vi "DB - [MasterData].[Material].vi"(0 "connection reference":T5, 1 "DB Connection":T2={"Open"=TRUE, "Close"=TRUE}, 2 "DB - Master Data Material Enum":T4, 3 "Include Inactive":bool=TRUE, 5 "SRTRS.MasterData.SAPMaterial/Material":string="SRTRS.MasterData.SAPMaterial", 7 "[LanguageId]":string, 9 "Update [ShortDescription] to Cluster":bool=TRUE, 11 "error in (no error)":errorcluster, 12 "Clust Refnum":refnum<vi>, 13 "Material File":path=path "c:/temp/Filestream/Test2.jpg", 14 "CmbBox Refnum":refnum<vi>) -> (4 "connection reference":T5, 6 "image data":T1, 8 "ImageFile OK":bool, 10 "Material File":path, 15 "SUMMARY":errorcluster)   [LabVIEW 2013]
uses:
  <vilib>/addons/database/Connection.llb/Conn ObjectReference.ctl
  Controls/DB - Master Data Material Enum.ctl
  Controls/DB - OpenClose.ctl
  <vilib>/picture/picture.llb/imagedata.ctl
  Controls/Global SRTRS.vi
  <vilib>/addons/database/Connection.llb/DB Tools Open Connec (String).vi
  <vilib>/addons/database/Connection.llb/Conn Execute.vi
  <vilib>/addons/database/Recordset.llb/Rec Fetch Recordset Data (R).vi
  <vilib>/addons/database/Recordset.llb/Rec Destroy - Connection.vi
  <vilib>/addons/database/_DB Variant To Data/Database Variant To Data.xnode
  <vilib>/addons/database/NI_Database_API.lvlib
panel:
  in  "SRTRS.MasterData.Material":string="SRTRS.MasterData.Material"
  out "JPG File Error":errorcluster
  out "Property Node Error":errorcluster
  out "Close Error":errorcluster
  out "ImageFileType":string
  out "Results":string[](array[string])
  in  "Material":T3 caption="Header"
  out "ms":u32
  out "SQL Query":errorcluster
  out "SQL":string="Use [SRTRS]\n\nIF NOT EXISTS(SELECT 1 from [MasterData].[Material]\nWHERE [MaterialNo] = 'M101' AND [MaterialRev]= '2' AND [LanguageId] = '' )\n\nBEGIN\nINSERT INTO [MasterData].[Material]\n           ([MaterialNo],[MaterialRev],[LanguageId])\nVALUES\n           ('M101', '2','')\nEND\n\n\nUPDATE [MasterData].[Material]\nSET [MaterialNo] = 'M101'  ,[MaterialRev] = '2'  ,[Description] = ''  ,[imageFilePath] = 'c:\\temp\\SRTRS4070\\MasterData\\JPG'  ,[ImageFileName] = 'M101_2.jpg'  ,[Inactive] = '0'  \nWHERE  [MaterialNo] = 'M101' AND [MaterialRev]= '2' AND [LanguageId] = '' \n"
  out "Connection Information":T6={"Connection "="SQL Server 32bit HPEnvy", "Username"="admin", "Password"="admin123"}
  # "imagedata.ctlDECLARE @image1    VARBINARY(MAX)\nSELECT @image1 = CAST(bulkcolumn AS VARBINARY(MAX))\n\nFROM OPENROWSET(BULK 'C:\\temp\\Filestream\\test1.jpg', SINGLE_BLOB) AS x\n\nUpdate T1 \nSET MyFile = @image1\nWHERE Msgid = 6;"
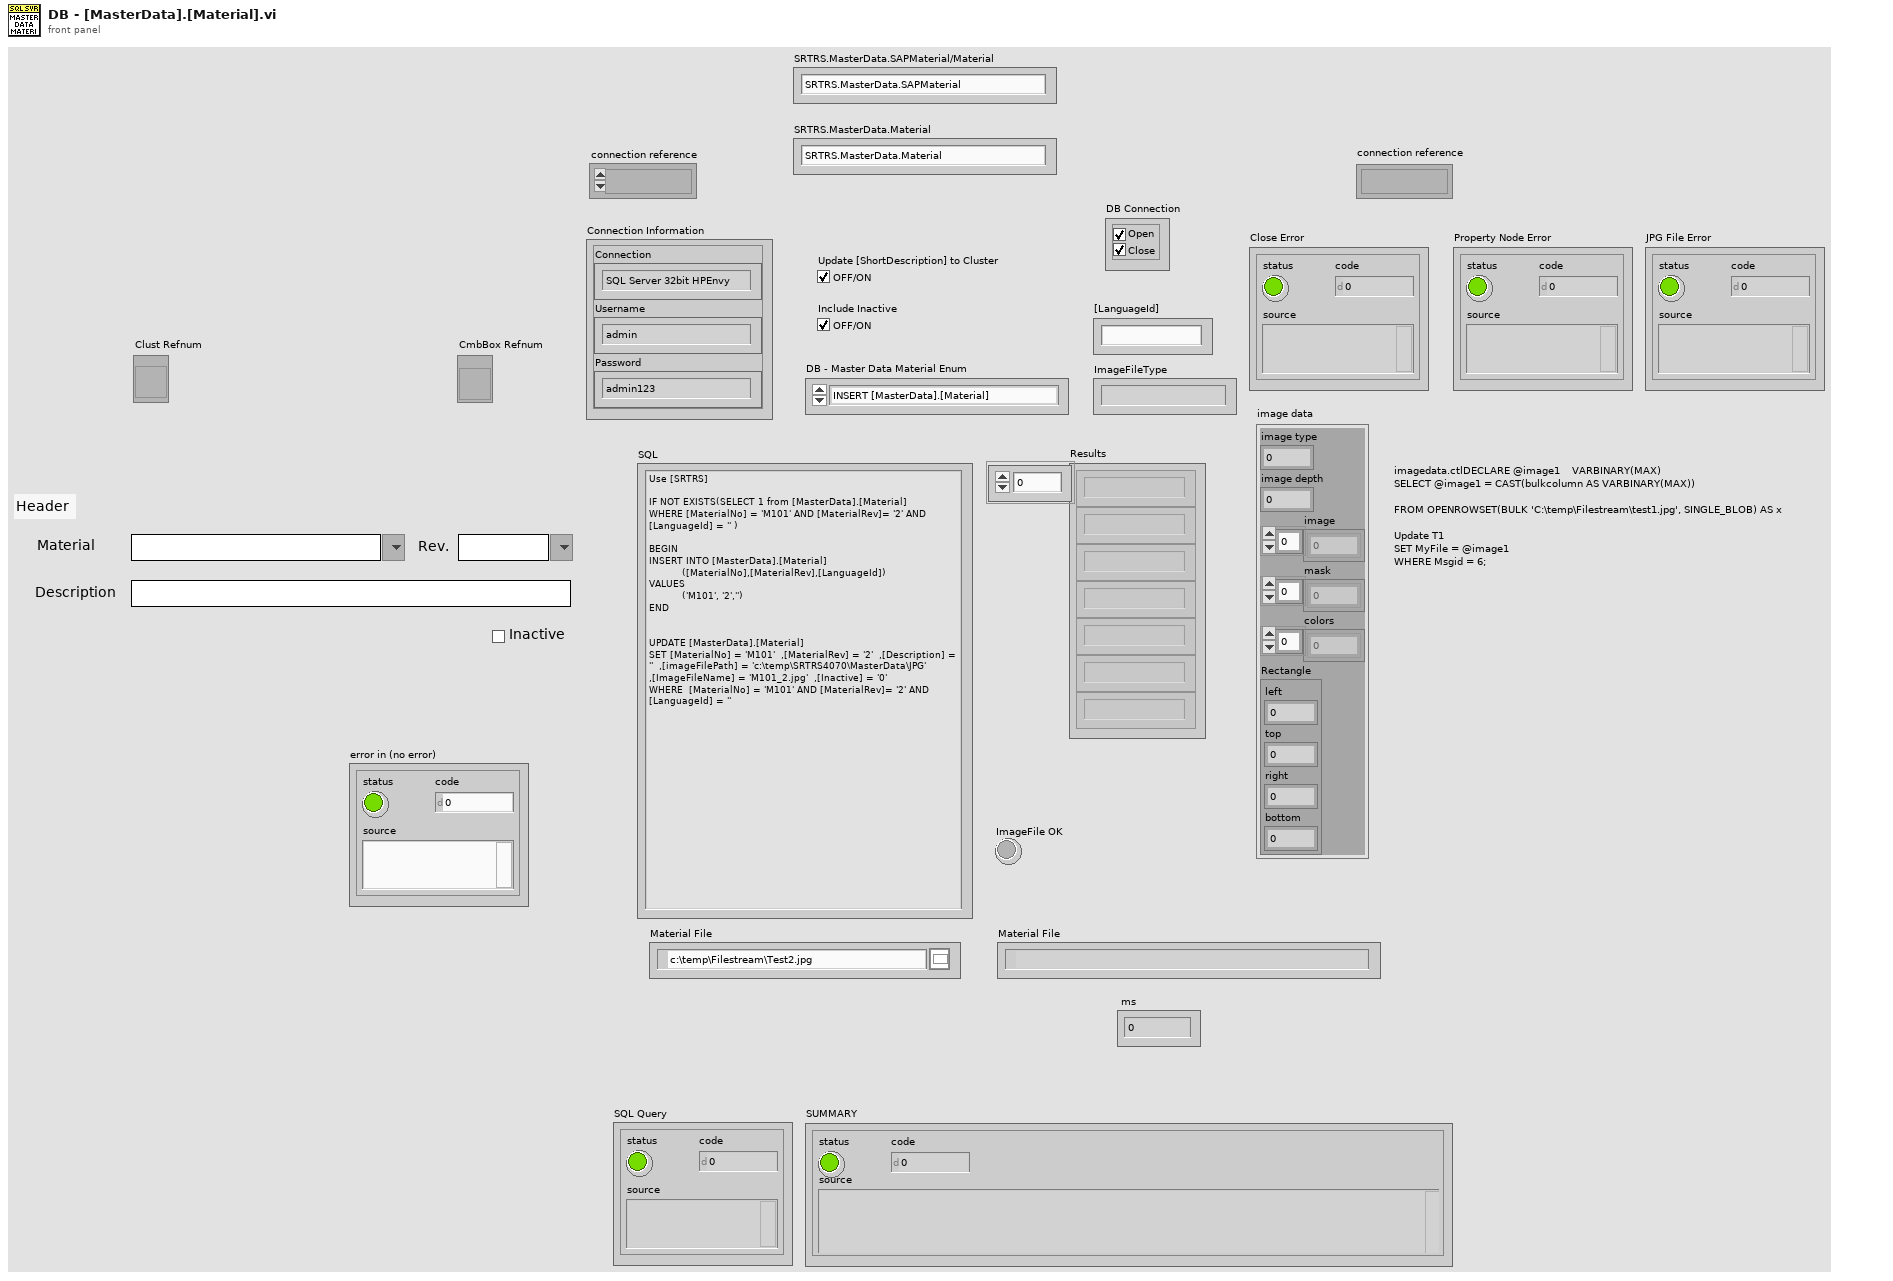
[diagram p1: front panel]
types:
  T1 = typedef "imagedata.ctl" = cluster{"image type":i32, "image depth":i32, "image":u8[], "mask":u8[], "colors":u32[], "Rectangle":cluster{"left":i16, "top":i16, "right":i16, "bottom":i16}}
  T2 = typedef "DB - OpenClose.ctl" = cluster{"Open":bool, "Close":bool}
  T3 = cluster{"Master Data Material":string, "Master Data Rev":string, "Master Data Material Description":string, "Inactive":bool}
  T4 = typedef "DB - Master Data Material Enum.ctl" = enum16{"INSERT [MasterData].[Material]", "UPDATE [MasterData].[Material]", "SELECT [MaterialNo]", "SELECT [ShortDescription]", "SELECT [MaterialRev]", "SELECT [Description], [ImageFile]", "SELECT [Description] (Long)"}
  T5 = typedef "NI_Database_API.lvlib/Conn ObjectReference.ctl" = refnum<k1>
  T6 = cluster{"Connection ":string, "Username":string, "Password":string}
  T7 = typedef "Enum - InteractiveMode-SubVIMode.ctl" = enum16{"Interactive", "subVI Mode"}
  T8 = typedef "DB - Logon Extra Info.ctl" = cluster{"Plant Name":string, "UserName":string, "Hostname [ClientName]":string, "IsUnicode":bool}
  T9 = typedef "Connection Information Cluster.ctl" = cluster{"Connection ":string, "Username":string, "Password":string}
  T10 = typedef "DB - DB.Schema.Table.ctl" = cluster{"DB":string, "Schema":string, "Table":string}
  T11 = typedef "NI_Database_API.lvlib/Rec ObjectReference.ctl" = refnum<k1>
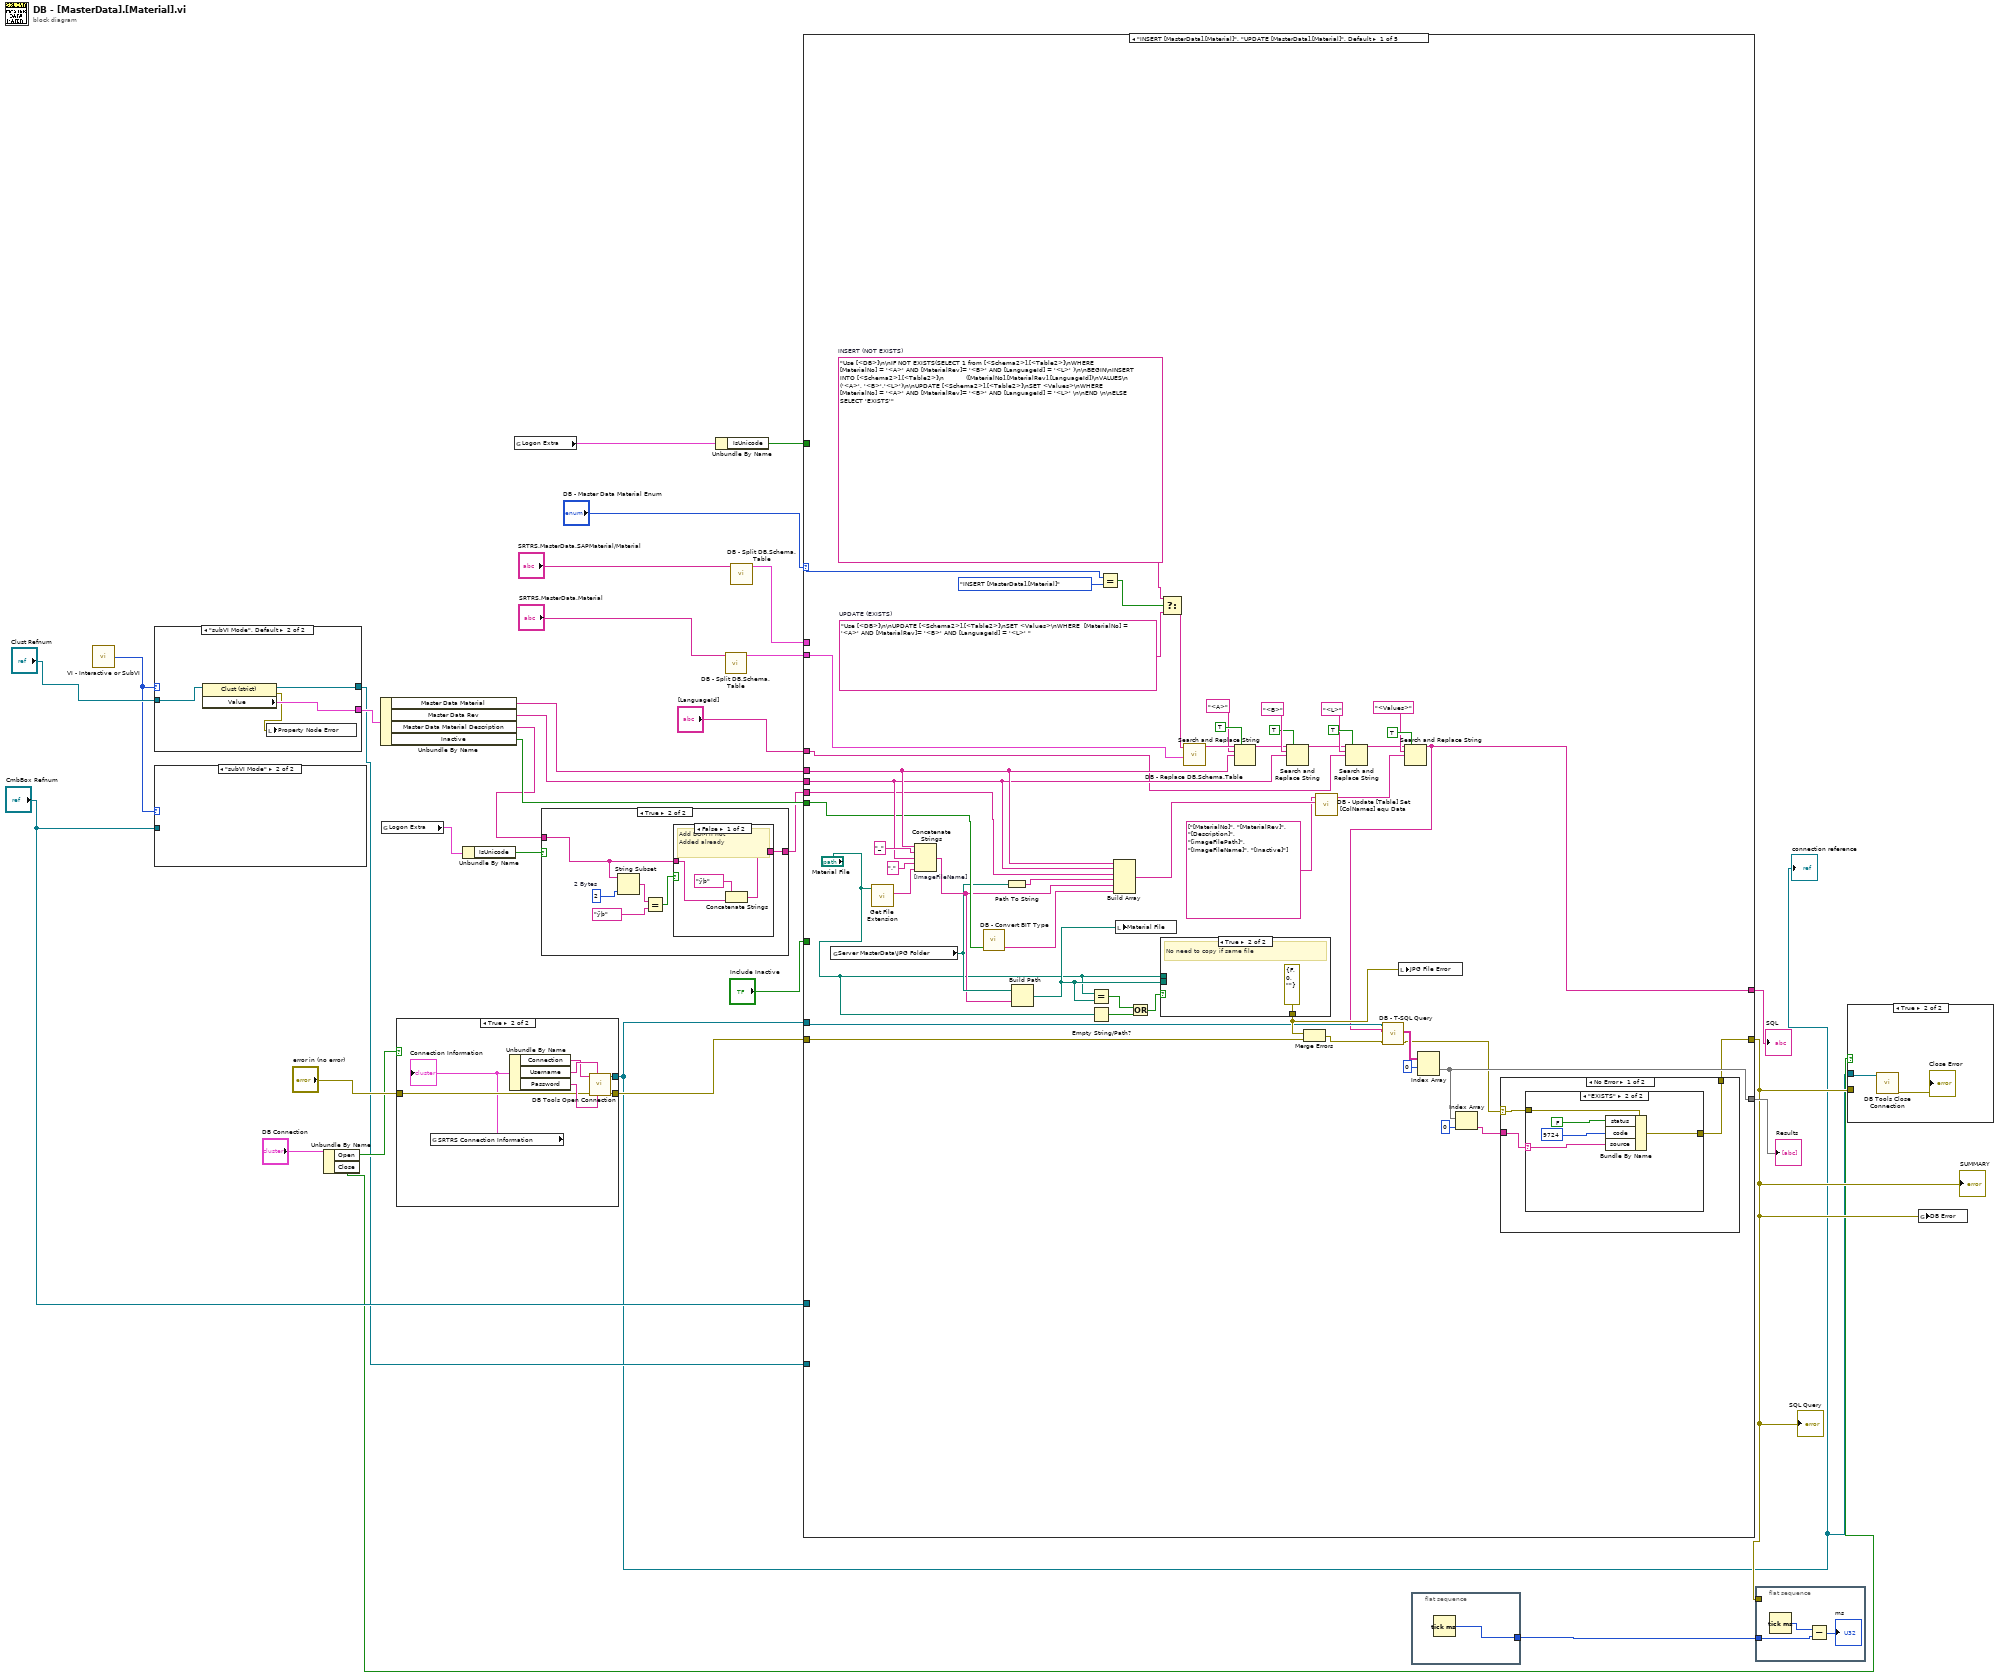
[diagram p0: block diagram]
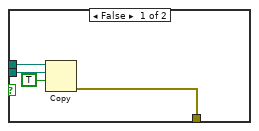
[diagram p7: hidden frame]
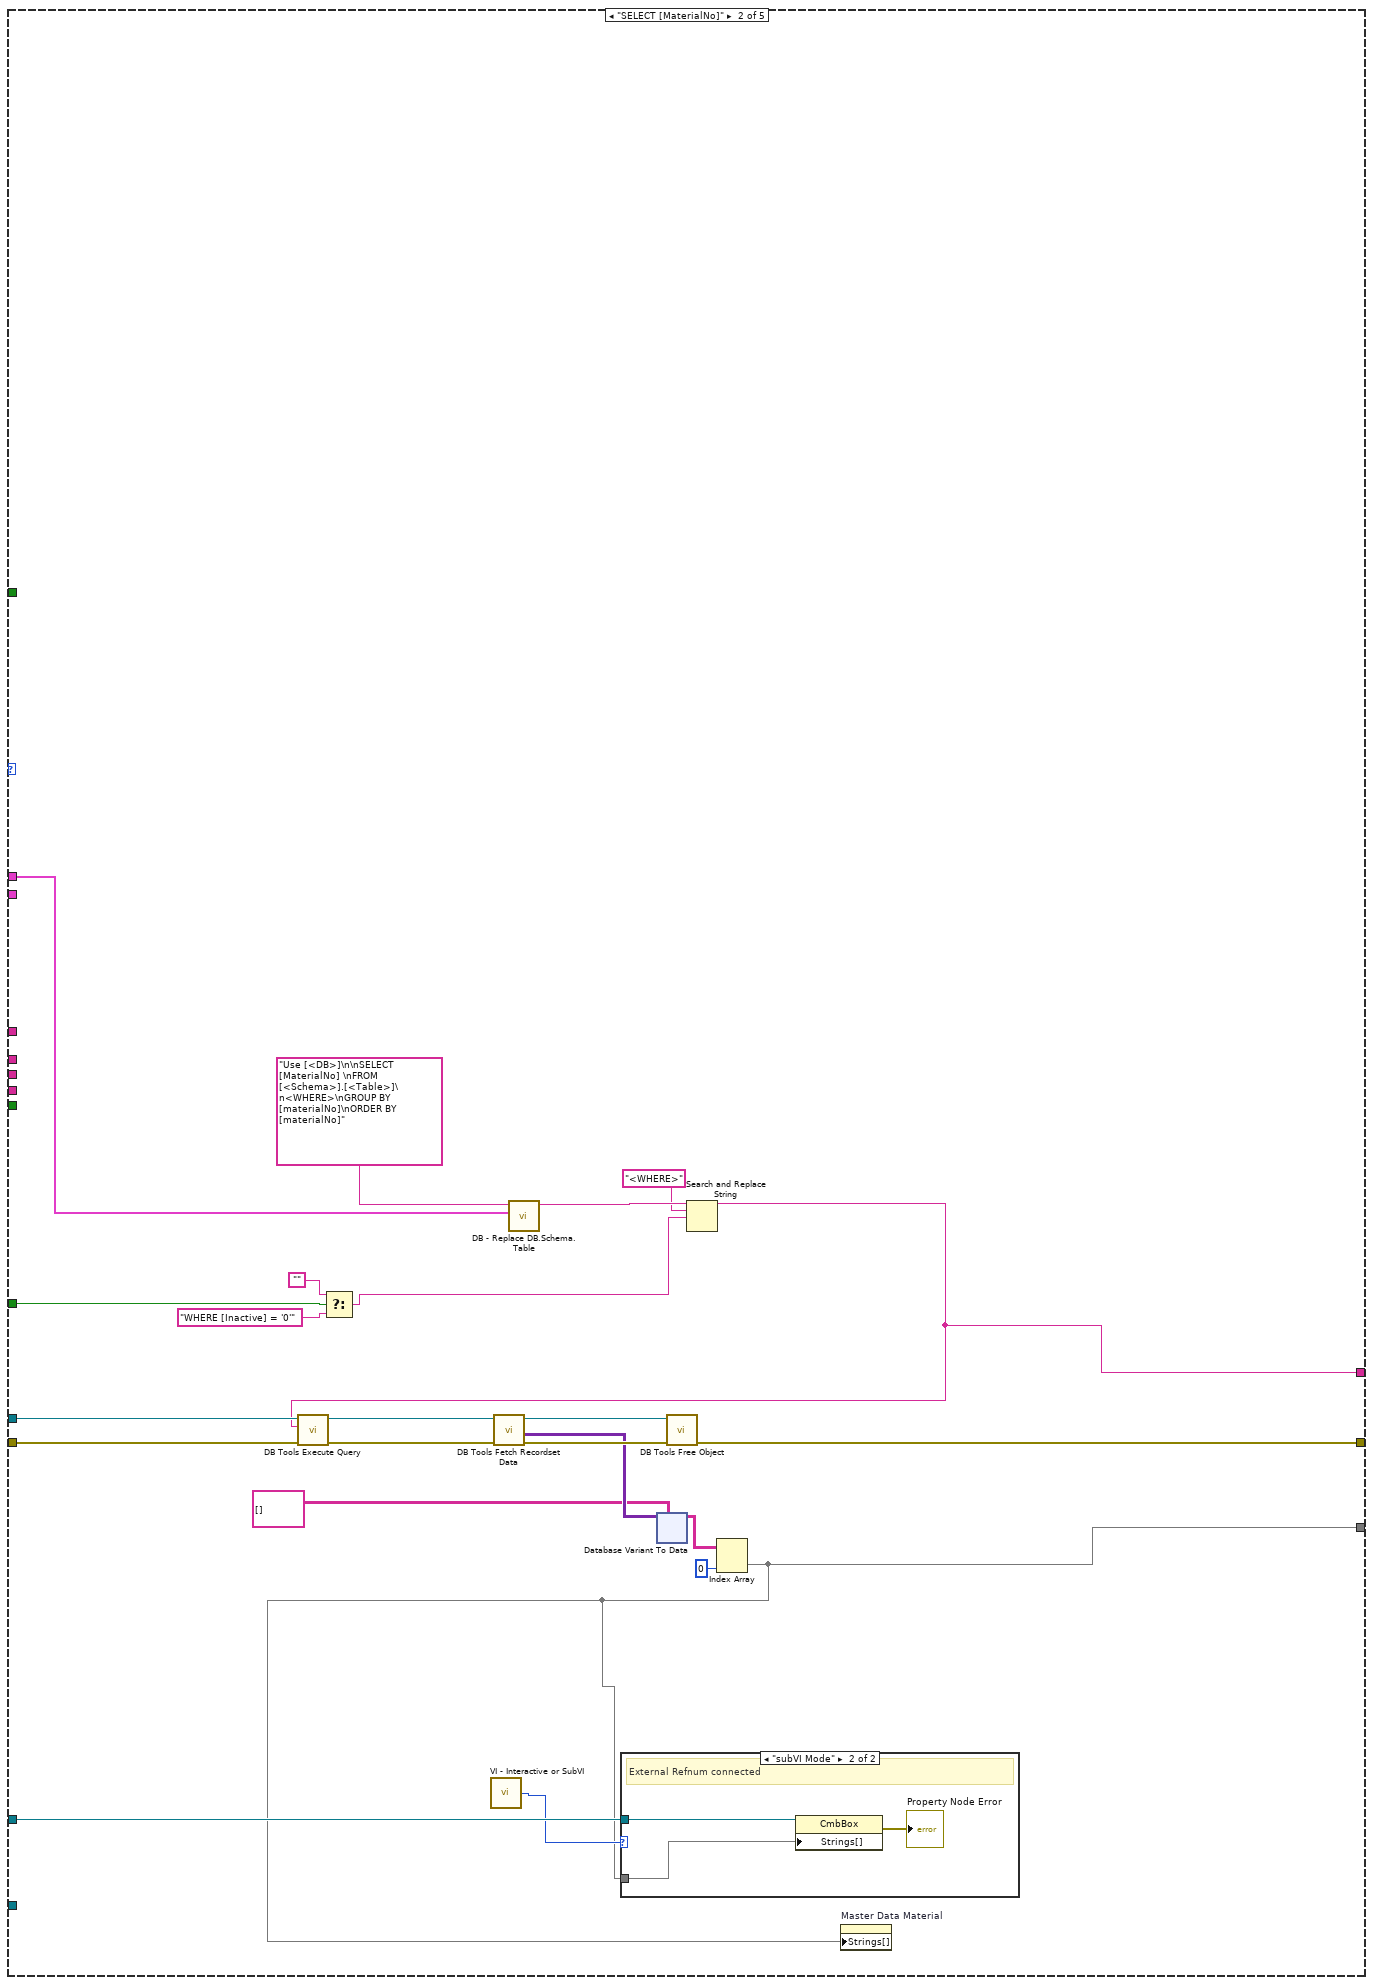
[diagram p8: hidden frame]
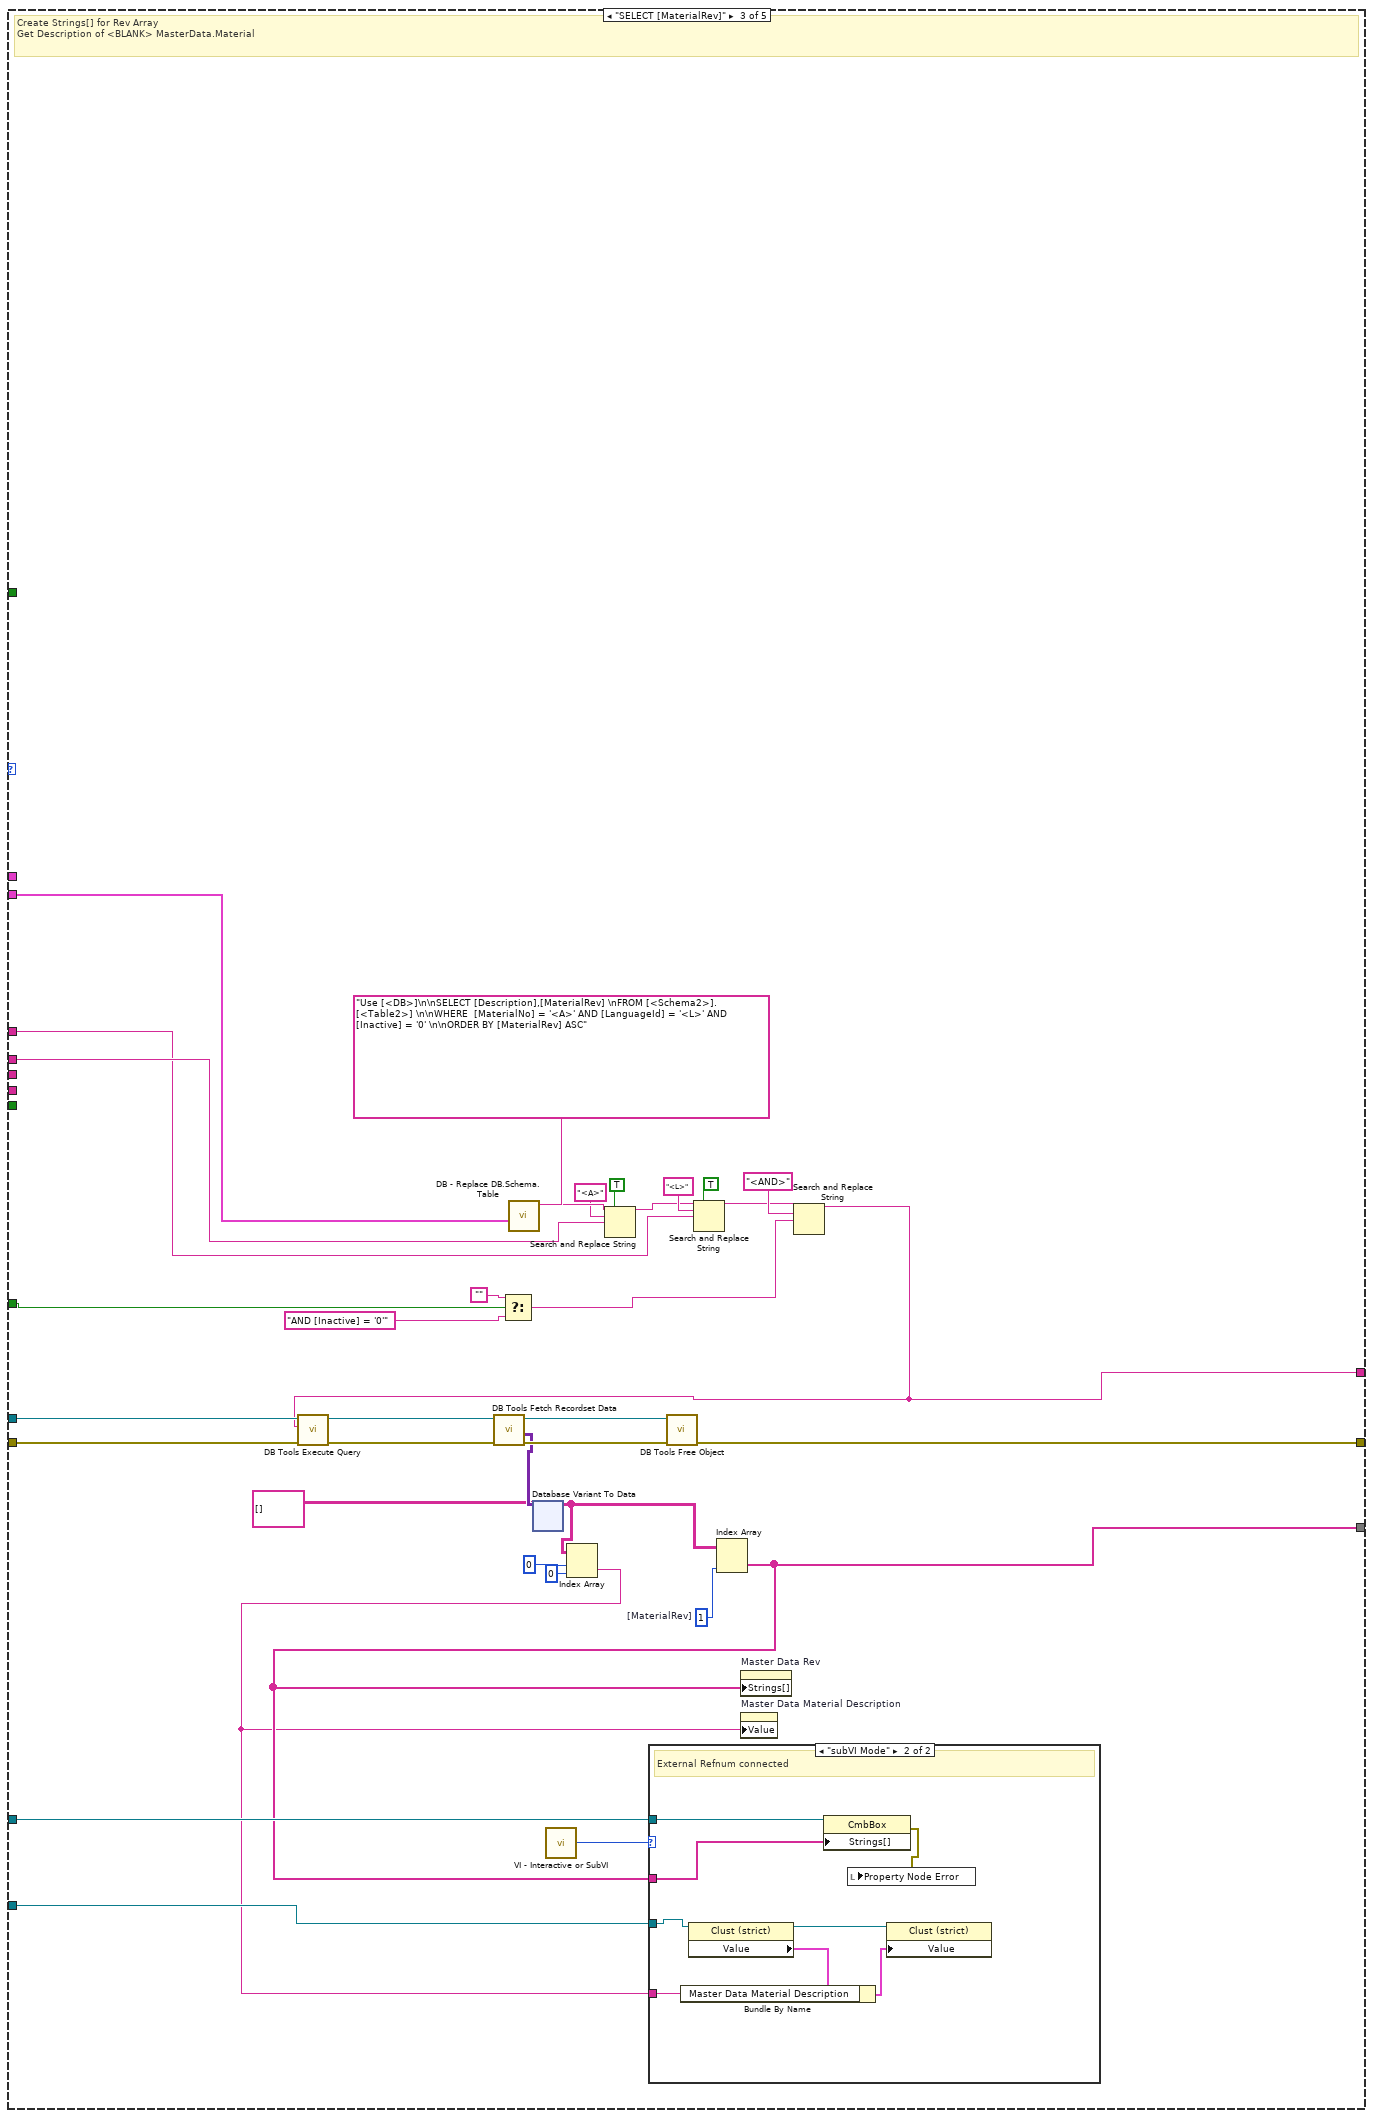
[diagram p10: hidden frame]
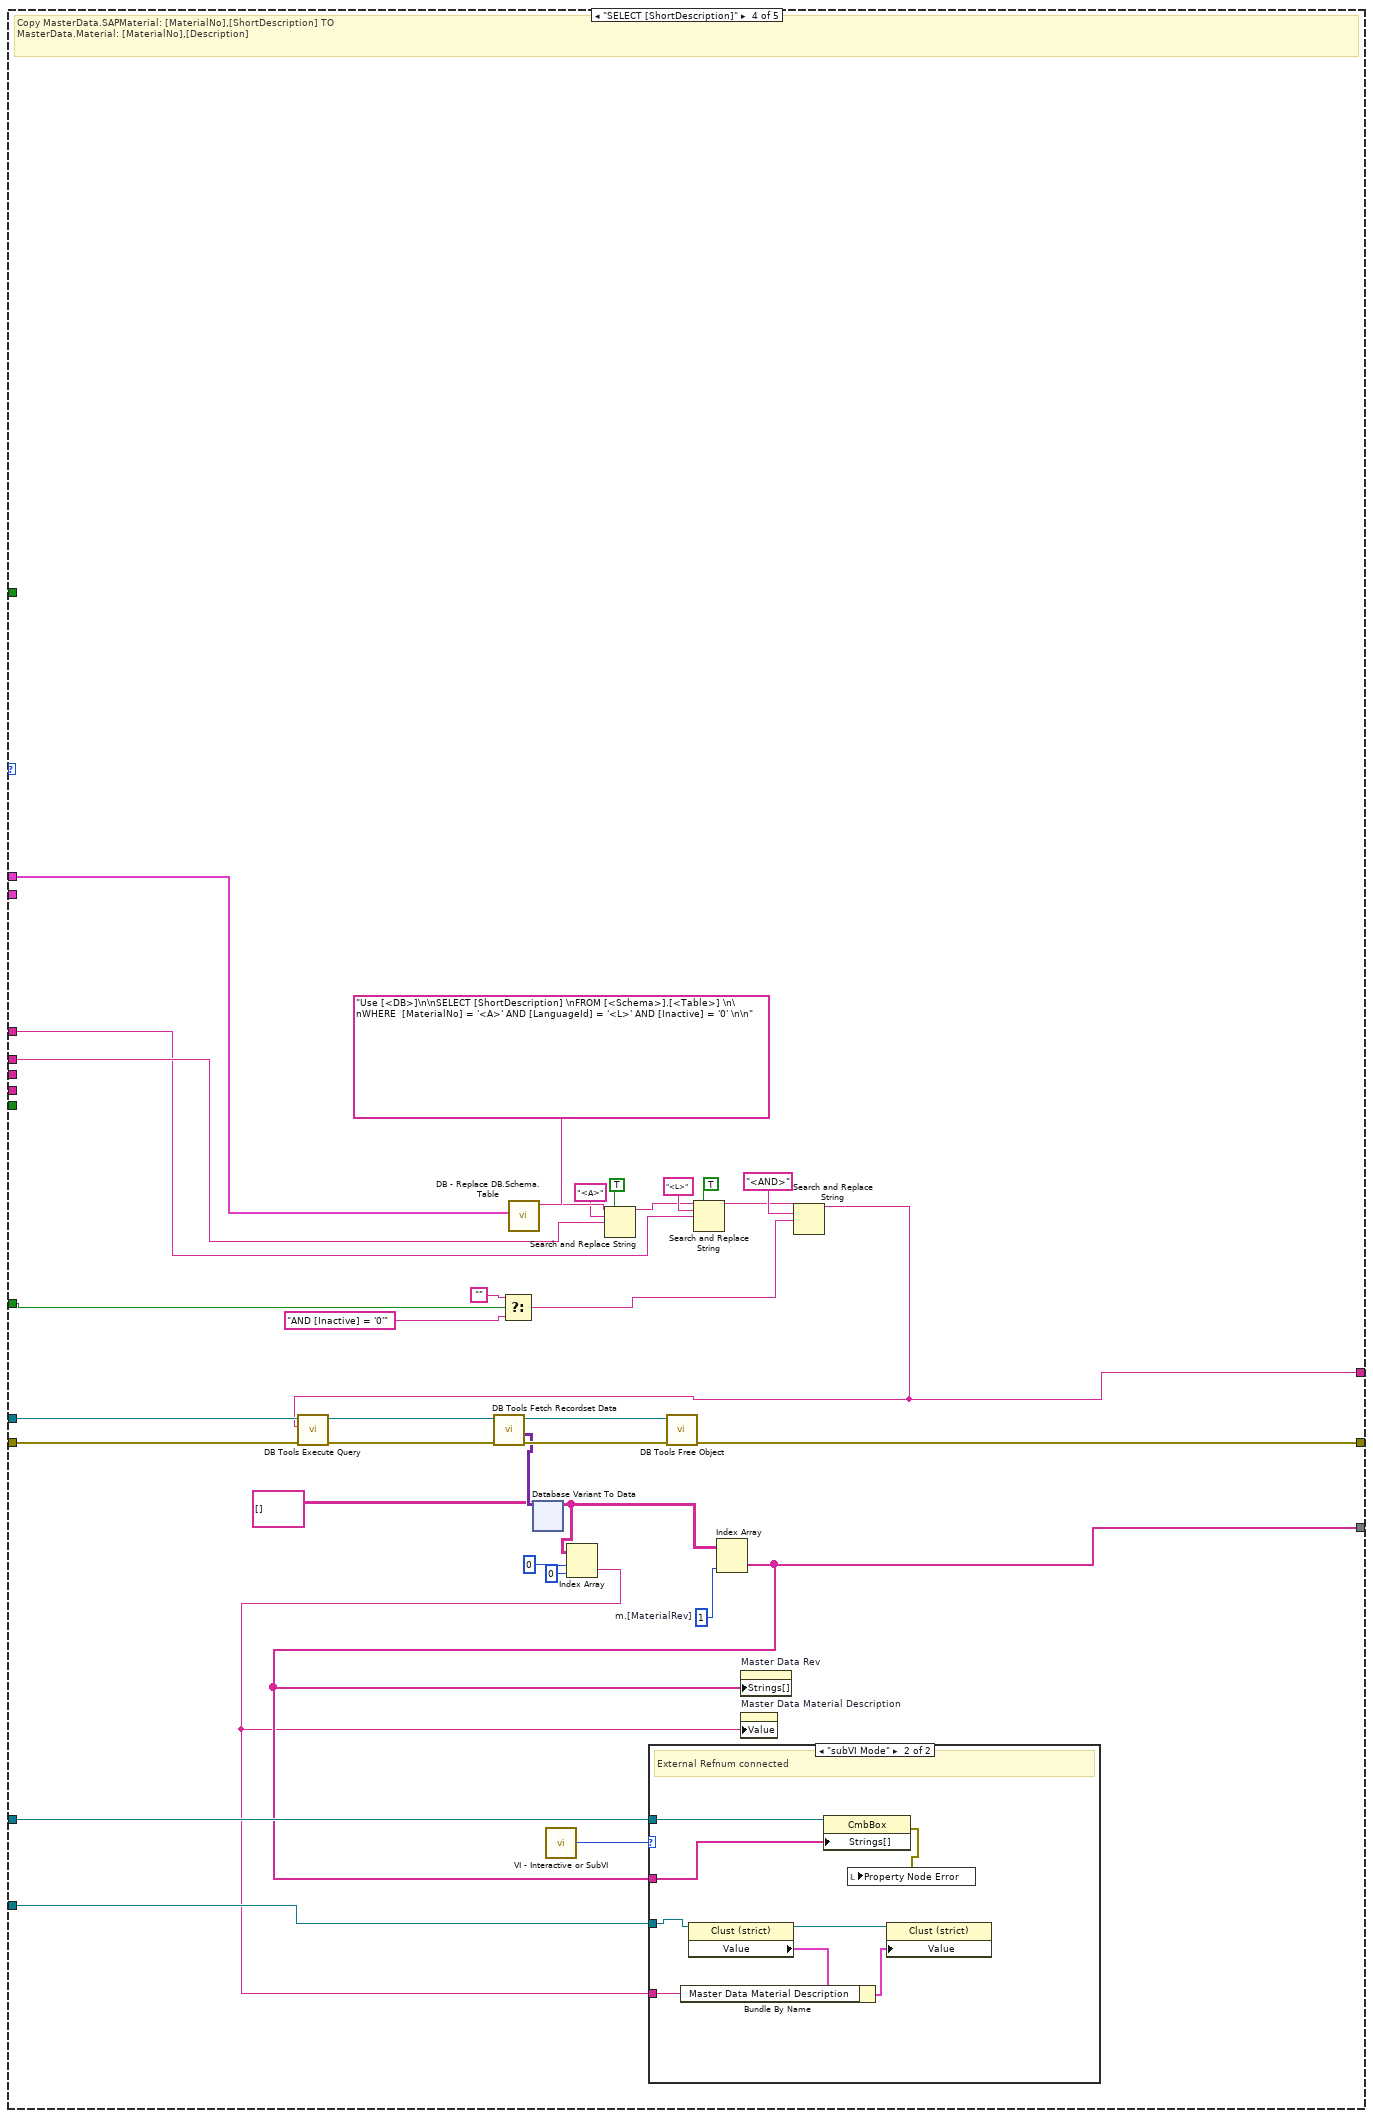
[diagram p12: hidden frame]
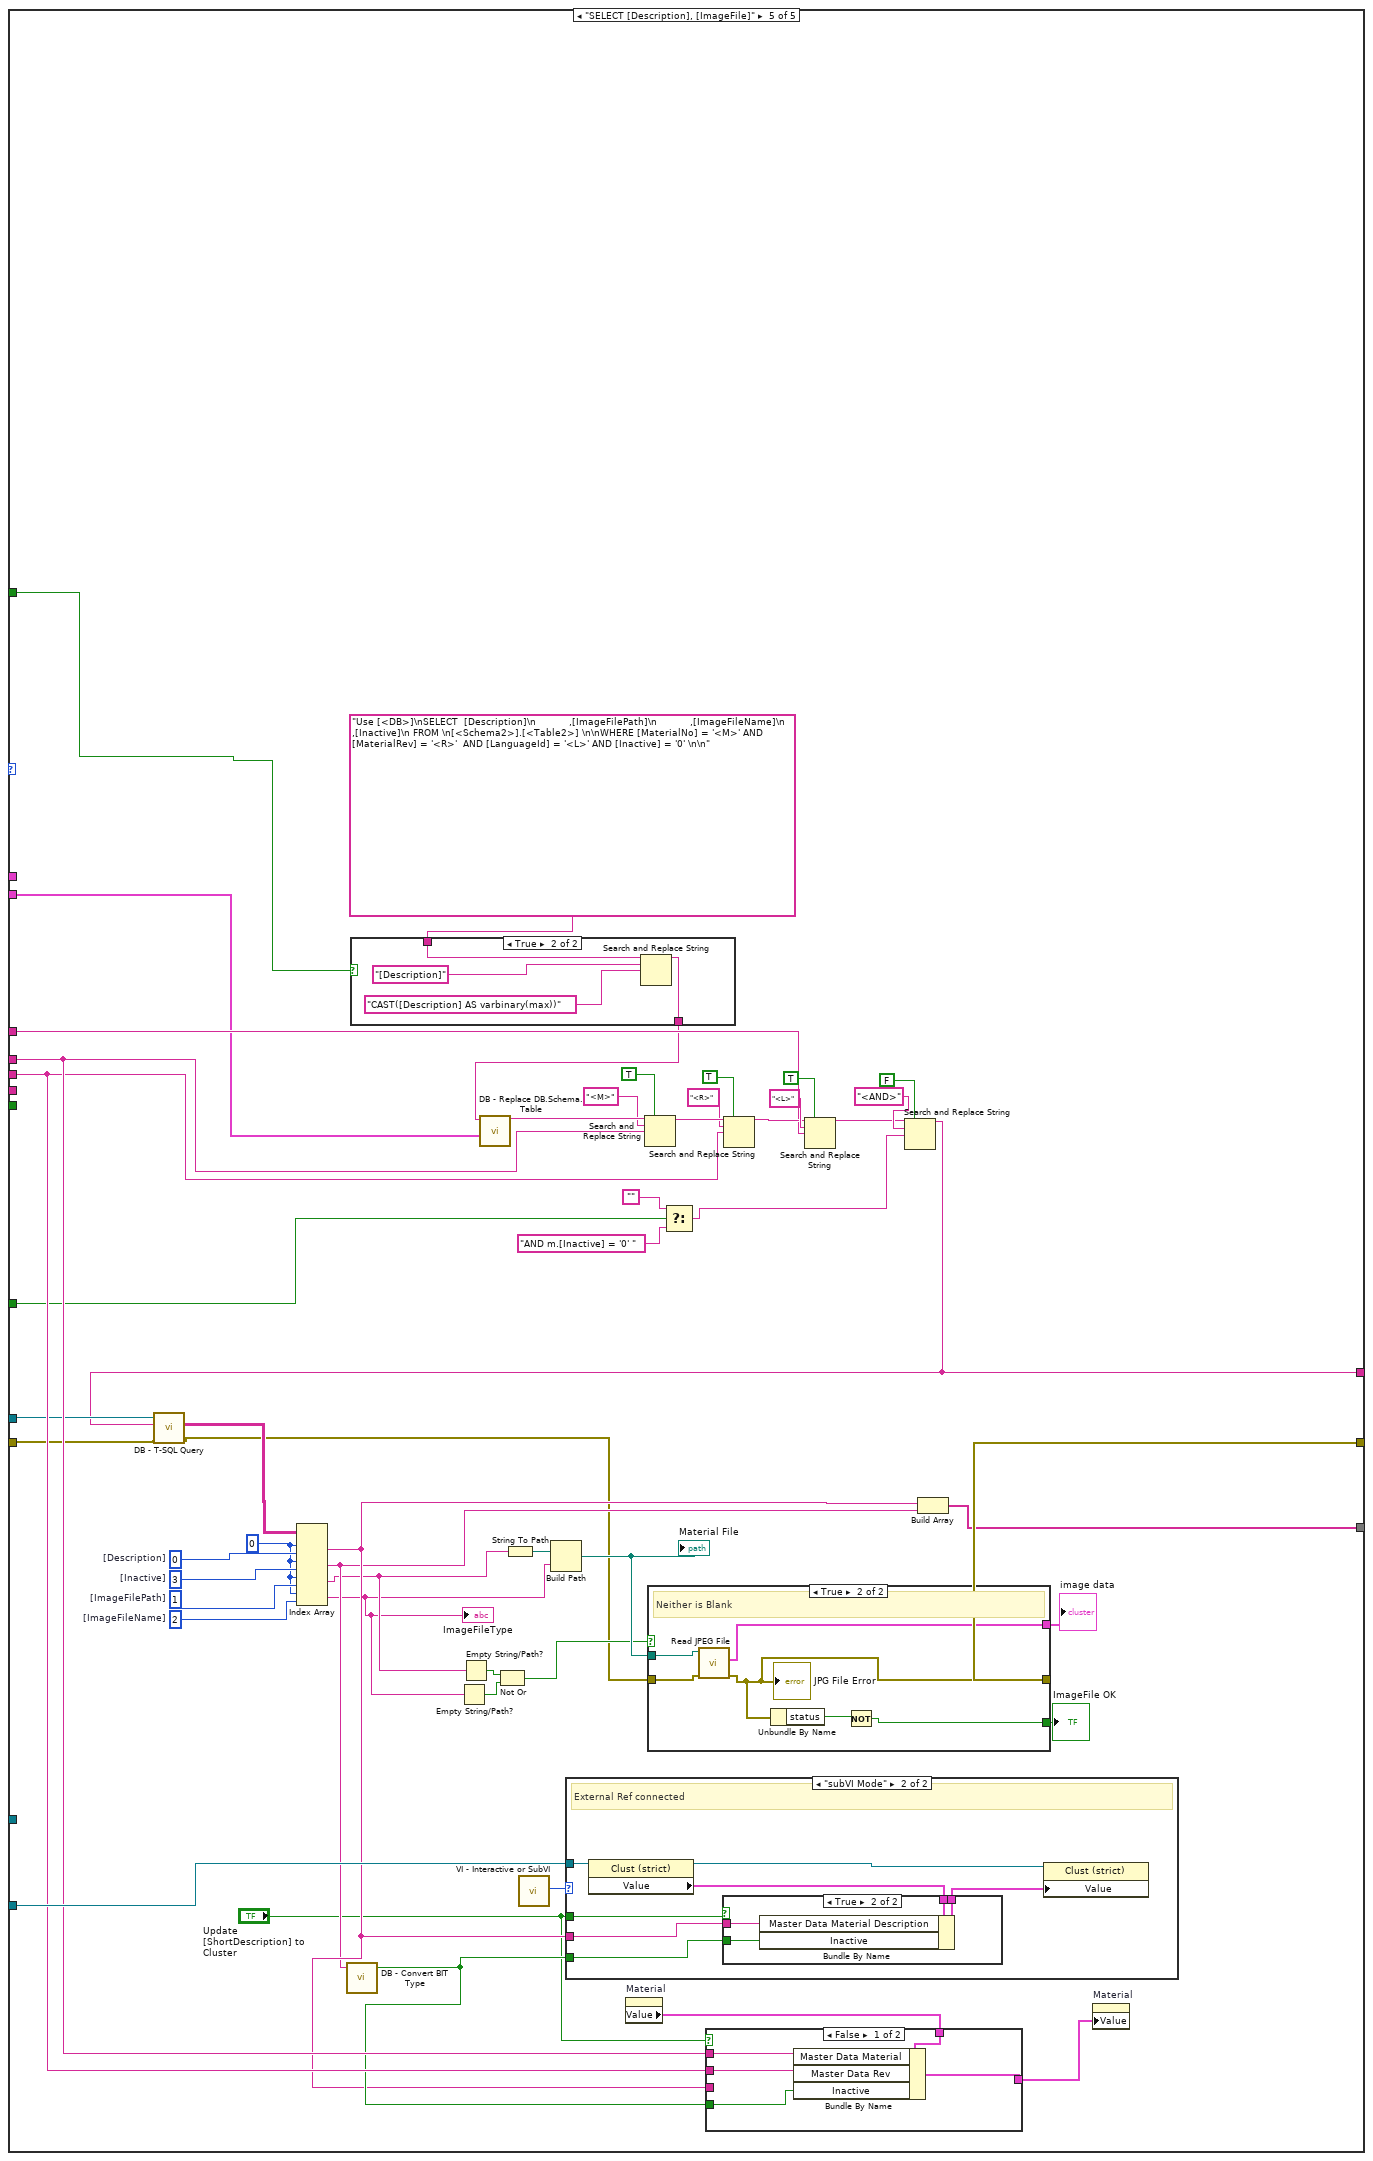
[diagram p14: hidden frame]
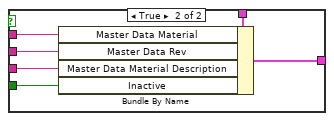
[diagram p16: hidden frame]
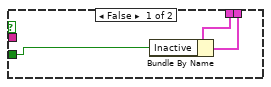
[diagram p19: hidden frame]
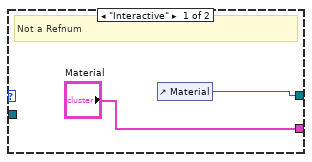
[diagram p20: hidden frame]
diagram:
  n1 = call "VI - Interactive or SubVI.vi"() -> ("Mode"=w15:T7)  [unwired: 5 in]
  n2 = case shown="\"subVI Mode\", Default" w15 {
    tunnel: "Clust Refnum" -> [_ w37]
    tunnel: ["Material" w36] -> w28
    tunnel: [w32 w35] -> w14
    frame "Interactive" {
      # "Not a Refnum"
      n3 = control-ref of="Material"() -> (w32:refnum<vi>)
    }
    frame "subVI Mode", Default {
      n4 = property class="Clust (strict)"(reference=w37) -> (reference out=w35:refnum<vi>, error out=w34:errorcluster, "Value"=w36:T3)  [unwired: 1 in]
      n5 = local write "Property Node Error"(w34) -> ()
    }
  }
  n6 = case shown="\"subVI Mode\"" w15 {
    tunnel: "CmbBox Refnum" -> [_ _]
    frame "Interactive", Default {
    }
    frame "subVI Mode" {
    }
  }
  n7 = Unbundle By Name("DB Connection") -> ("Open"=w17:bool, "Close"=w16:bool)
  n8 = Unbundle By Name(w28) -> ("Master Data Material"=w13:string, "Master Data Rev"=w12:string, "Master Data Material Description"=w2:string, "Inactive"=w11:bool)
  n9 = global read "Global SRTRS.vi" "Logon Extra"() -> (w4:T8)
  n10 = case shown="True" w17 {
    tunnel: ["connection reference" w43] -> w7
    tunnel: "error in (no error)" -> [w38 w42]
    tunnel: [w38 w41] -> w25
    frame False {
      # "subVI"
    }
    frame True {
      n11 = global read "Global SRTRS.vi" "SRTRS Connection Information"() -> (w40:T9)
      "Connection Information" <- w40
      n12 = Unbundle By Name(w40) -> ("Connection"=w45:string, "Username"=w46:string, "Password"=w44:string)
      n13 = call-poly <vilib>:"DB Tools Open Connection.vi"("password"=w44, "userID"=w46, "error in (no error)"=w42, "connection information"=w45) -> ("error out"=w41:errorcluster, "connection reference"=w43:T5)  [unwired: 4 in]
    }
  }
  "connection reference" <- w7
  n14 = Unbundle By Name(w4) -> ("IsUnicode"=w3:bool)
  n15 = global read "Global SRTRS.vi" "Logon Extra"() -> (w6:T8)
  n16 = case shown="True" w3 {
    tunnel: w2 -> [w47 w50]
    tunnel: [w47 w48] -> w1
    frame False {
    }
    frame True {
      w53 = 2  # 2 Bytes
      n17 = String Subset(string=w50, length (rest)=w53) -> (substring=w52:string)  [unwired: 1 in]
      n18 = Equal?(x=w52, y="ÿþ" ("search string")) -> (x = y?=w49:bool)
      n19 = case shown="False" w49 {
        tunnel: w50 -> [w56 w57]
        tunnel: [w54 w57] -> w48
        frame False {
          # "Add BOM if not \nAdded already"
          n20 = Concatenate Strings("ÿþ", w56) -> (w54:string)
        }
        frame True {
        }
      }
    }
  }
  n21 = Unbundle By Name(w6) -> ("IsUnicode"=w5:bool)
  n22 = call "DB - Split DB.Schema.Table.vi"("DB.Schema.Table"="SRTRS.MasterData.Material") -> ("DB.Schema.Table"=w9:T10)  [unwired: 10 in]
  n23 = call "DB - Split DB.Schema.Table.vi"("DB.Schema.Table"="SRTRS.MasterData.SAPMaterial/Material") -> ("DB.Schema.Table"=w29:T10)  [unwired: 10 in]
  n24 = case shown="\"INSERT [MasterData].[Material]\", \"UPDATE [MasterData].[Material]\", Default" "DB - Master Data Material Enum" {
    selector: "DB - Master Data Material Enum" -> [w69 _ _ _ _]
    tunnel: w7 -> [w77 w146 w228 w315 w373]
    tunnel: [w62 w144 w226 w313 w419] -> w19
    tunnel: w29 -> [_ w142 _ w286 _]
    tunnel: w13 -> [w95 _ w212 w299 w406]
    tunnel: w12 -> [w94 _ _ _ w405]
    tunnel: [w75 w132 w208 w295 w372] -> w27
    tunnel: w25 -> [w89 w145 w227 w314 w371]
    tunnel: [w66 w124 w216 w303 w410] -> w23
    tunnel: "CmbBox Refnum" -> [_ w134 w217 w304 _]
    tunnel: w14 -> [_ _ w198 w285 w409]
    tunnel: "Include Inactive" -> [_ w131 w206 w293 w396]
    tunnel: w1 -> [w93 _ _ _ _]
    tunnel: w11 -> [w92 _ _ _ _]
    tunnel: w9 -> [w78 _ w199 _ w376]
    tunnel: "[LanguageId]" -> [w79 _ w200 w287 w378]
    tunnel: w5 -> [_ _ _ _ w369]
    frame "INSERT [MasterData].[Material]", "UPDATE [MasterData].[Material]", Default {
      w71 = "Use [<DB>]\n\nUPDATE [<Schema2>].[<Table2>]\nSET <Values>\nWHERE  [MaterialNo] = '<A>' AND [MaterialRev]= '<B>' AND [LanguageId] = '<L>' "  # UPDATE (EXISTS)
      w72 = "Use [<DB>]\n\nIF NOT EXISTS(SELECT 1 from [<Schema2>].[<Table2>]\nWHERE [MaterialNo] = '<A>' AND [MaterialRev]= '<B>' AND [LanguageId] = '<L>' )\n\nBEGIN\nINSERT INTO [<Schema2>].[<Table2>]\n           ([MaterialNo],[MaterialRev],[LanguageId])\nVALUES\n           ('<A>', '<B>','<L>')\n\nUPDATE [<Schema2>].[<Table2>]\nSET <Values>\nWHERE  [MaterialNo] = '<A>' AND [MaterialRev]= '<B>' AND [LanguageId] = '<L>' \n\nEND \n\nELSE SELECT 'EXISTS'"  # INSERT (NOT EXISTS)
      n25 = global read "Global SRTRS.vi" "Server MasterData\\JPG Folder"() -> (w91:path)
      n26 = call <vilib>:"Get File Extension.vi"("file"="Material File") -> ("lowercase file extension"=w99:string)  [unwired: 7 in, 3 out]
      n27 = Concatenate Strings "[ImageFileName]"(w95, "_" ("string"), w94, "." ("string"), w99) -> (w90:string)
      n28 = call "DB - Convert BIT Type.vi"("Boolean"=w92) -> ("BIT (eg Inactive)"=w96:string)  [unwired: 2 in, 2 out]
      n29 = Path To String(path=w91) -> (string=w100:string)
      n30 = Build Path(base path=w91, name or relative path=w90) -> (appended path=w88:path)
      n31 = Equal?(x="Material File", y=w88) -> (x = y?=w60:bool)
      n32 = Empty String/Path?(string/path="Material File") -> (empty?=w59:bool)
      n33 = Equal?(x=w69, y=DB_-_Master_Data_Material_Enum."INSERT [MasterData].[Material]") -> (x = y?=w67:bool)
      n34 = Build Array(w95, w94, w93, w100, w90, w96) -> (w86:string[])
      n35 = local write "Material File"(w88) -> ()
      n36 = Or(x=w60, y=w59) -> (x .or. y?=w58:bool)
      n37 = case shown="True" w58 {
        tunnel: [w121 errorcluster {"status"=FALSE, "code"=0, "source"=""} ("error out")] -> w87
        tunnel: "Material File" -> [w120 _]
        tunnel: w88 -> [w119 _]
        frame False {
          n38 = Copy(9:TRUE ("overwrite (F)"), 10:w119, 11:w120) -> (0:w121:errorcluster)  [unwired: 2 in, 2 out]
        }
        frame True {
          # "No need to copy if same file"
        }
      }
      n39 = Select(t=w72, s=w67, f=w71) -> (s? t:f=w70:string)
      n40 = call "DB - Replace DB.Schema.Table.vi"("DB.Schema.Table 2"=w78, "string in"=w70) -> ("string out"=w107:string)  [unwired: 8 in, 1 out]
      n41 = Search and Replace String(replace all?=TRUE ("replace all? (F)"), input string=w107, search string="<A>", replace string=w95) -> (result string=w103:string)  [unwired: 4 in, 3 out]
      n42 = Search and Replace String(replace all?=TRUE ("replace all? (F)"), input string=w103, search string="<B>", replace string=w94) -> (result string=w81:string)  [unwired: 4 in, 3 out]
      n43 = Merge Errors(w87, w89) -> (w76:errorcluster)
      n44 = call "DB - Update [Table] Set [ColNames] equ Data.vi"("<Data> (0xFFFE autodetect)"=w86, "[ColumnNames]"=string[] ["[MaterialNo]", "[MaterialRev]", "[Description]", "[imageFilePath]", "[ImageFileName]", "[Inactive]"]) -> ("<Values>"=w84:string)  [unwired: 9 in]
      n45 = Search and Replace String(replace all?=TRUE ("replace all? (F)"), input string=w81, search string="<L>", replace string=w79) -> (result string=w80:string)  [unwired: 4 in, 3 out]
      n46 = local write "JPG File Error"(w87) -> ()
      n47 = Search and Replace String(replace all?=TRUE ("replace all? (F)"), input string=w80, search string="<Values>", replace string=w84) -> (result string=w75:string)  [unwired: 4 in, 3 out]
      n48 = call "DB - T-SQL Query.vi"("error in (no error)"=w76, "T-SQL"=w75, "connection reference"=w77) -> ("error out"=w64:errorcluster, "2D data"=w74:string[][])  [unwired: 6 in, 1 out]
      n49 = Index Array(array=w74, index (row)=0) -> (element=w66:string[])  [unwired: 1 in]
      n50 = Index Array(array=w66, index=0) -> (element=w63:string)
      n51 = case shown="No Error" w64 {
        selector: w64 -> [w111 w118]
        tunnel: w63 -> [w109 _]
        tunnel: [w110 w118] -> w62
        frame No Error {
          n52 = case shown="\"EXISTS\"" w109 {
            selector: w109 -> [_ w113]
            tunnel: w111 -> [w112 w117]
            tunnel: [w112 w116] -> w110
            frame "False", Default {
            }
            frame "EXISTS" {
              n53 = Bundle By Name(cluster=w117, "status"=FALSE, "code"=9724, "source"=w113) -> (w116:errorcluster)
            }
          }
        }
        frame Error {
        }
      }
    }
    frame "SELECT [MaterialNo]" {
      n54 = Select(t="", s=w131, f="WHERE [Inactive] = '0'") -> (s? t:f=w129:string)
      n55 = call "VI - Interactive or SubVI.vi"() -> ("Mode"=w126:T7)  [unwired: 5 in]
      n56 = call "DB - Replace DB.Schema.Table.vi"("DB.Schema.Table"=w142, "string in"="Use [<DB>]\n\nSELECT [MaterialNo] \nFROM [<Schema>].[<Table>]\n<WHERE>\nGROUP BY [materialNo]\nORDER BY [materialNo]") -> ("string out"=w133:string)  [unwired: 8 in, 1 out]
      n57 = Search and Replace String(input string=w133, search string="<WHERE>", replace string=w129) -> (result string=w132:string)  [unwired: 5 in, 3 out]
      n58 = call-poly <vilib>:"DB Tools Execute Query.vi"("error in (no error)"=w145, "SQL query"=w132, "connection reference"=w146) -> ("error out"=w140:errorcluster, "recordset reference"=w141:T11)  [unwired: 5 in]
      n59 = call-poly <vilib>:"DB Tools Fetch Recordset Data.vi"("error in (no error)"=w140, "recordset reference"=w141) -> ("error out"=w139:errorcluster, "recordset data"=w138:variant[][], "recordset reference out"=w136:T11)  [unwired: 3 in]
      n60 = xnode "Database Variant To Data"("database variant"=w138, "type"=string[][] []) -> ("data"=w125:string[][])  [unwired: 1 in, 1 out]
      n61 = call-poly <vilib>:"DB Tools Free Object.vi"("error in (no error)"=w139, "recordset reference"=w136) -> ("error out"=w144:errorcluster)  [unwired: 8 in, 1 out]
      n62 = Index Array(array=w125, index (col)=0 ("disabled index (col)")) -> (element=w124:string[])  [unwired: 1 in]
      n63 = case shown="\"subVI Mode\"" w126 {
        tunnel: w134 -> [_ w149]
        tunnel: w124 -> [_ w148]
        frame "Interactive", Default {
          # "Not a Refnum"
        }
        frame "subVI Mode" {
          # "External Refnum connected"
          n64 = property class="CmbBox"(reference=w149, "Strings[]"=w148) -> (error out=→"Property Node Error":errorcluster)  [unwired: 1 in, 1 out]
        }
      }
      n65 = property on="Master Data Material" class="CmbBox"("Strings[]"=w124) -> ()  [unwired: 2 in, 2 out]
    }
    frame "SELECT [MaterialRev]" {
      w218 = 1  # [MaterialRev]
      # "Create Strings[] for Rev Array\nGet Description of <BLANK> MasterData.Material"
      n66 = Select(t="", s=w206, f="AND [Inactive] = '0'") -> (s? t:f=w211:string)
      n67 = call "DB - Replace DB.Schema.Table.vi"("DB.Schema.Table 2"=w199, "string in"="Use [<DB>]\n\nSELECT [Description],[MaterialRev] \nFROM [<Schema2>].[<Table2>] \n\nWHERE  [MaterialNo] = '<A>' AND [LanguageId] = '<L>' AND [Inactive] = '0' \n\nORDER BY [MaterialRev] ASC") -> ("string out"=w215:string)  [unwired: 8 in, 1 out]
      n68 = call "VI - Interactive or SubVI.vi"() -> ("Mode"=w205:T7)  [unwired: 5 in]
      n69 = Search and Replace String(replace all?=TRUE, input string=w215, search string="<A>", replace string=w212) -> (result string=w202:string)  [unwired: 4 in, 3 out]
      n70 = Search and Replace String(replace all?=TRUE, input string=w202, search string="<L>", replace string=w200) -> (result string=w201:string)  [unwired: 4 in, 3 out]
      n71 = Search and Replace String(input string=w201, search string="<AND>", replace string=w211) -> (result string=w208:string)  [unwired: 5 in, 3 out]
      n72 = call-poly <vilib>:"DB Tools Execute Query.vi"("error in (no error)"=w227, "SQL query"=w208, "connection reference"=w228) -> ("error out"=w223:errorcluster, "recordset reference"=w224:T11)  [unwired: 5 in]
      n73 = call-poly <vilib>:"DB Tools Fetch Recordset Data.vi"("error in (no error)"=w223, "recordset reference"=w224) -> ("error out"=w222:errorcluster, "recordset data"=w221:variant[][], "recordset reference out"=w219:T11)  [unwired: 3 in]
      n74 = xnode "Database Variant To Data"("database variant"=w221, "type"=string[][] []) -> ("data"=w197:string[][])  [unwired: 1 in, 1 out]
      n75 = Index Array(array=w197, index (row)=0, index (col)=0 ("disabled index (col)")) -> (element=w194:string)
      n76 = call-poly <vilib>:"DB Tools Free Object.vi"("error in (no error)"=w222, "recordset reference"=w219) -> ("error out"=w226:errorcluster)  [unwired: 8 in, 1 out]
      n77 = Index Array(array=w197, index (col)=w218) -> (element=w216:string[])  [unwired: 1 in]
      n78 = case shown="\"subVI Mode\"" w205 {
        tunnel: w217 -> [_ w236]
        tunnel: w216 -> [_ w235]
        tunnel: w198 -> [_ w233]
        tunnel: w194 -> [_ w229]
        frame "Interactive", Default {
          # "Not a Refnum"
        }
        frame "subVI Mode" {
          # "External Refnum connected"
          n79 = property class="Clust (strict)"(reference=w233) -> (reference out=w232:refnum<vi>, "Value"=w231:T3)  [unwired: 1 in, 1 out]
          n80 = Bundle By Name(cluster=w231, "Master Data Material Description"=w229) -> (w230:T3)
          n81 = property class="CmbBox"(reference=w236, "Strings[]"=w235) -> (error out=w234:errorcluster)  [unwired: 1 in, 1 out]
          n82 = local write "Property Node Error"(w234) -> ()
          n83 = property class="Clust (strict)"(reference=w232, "Value"=w230) -> ()  [unwired: 1 in, 2 out]
        }
      }
      n84 = property on="Master Data Rev" class="CmbBox"("Strings[]"=w216) -> ()  [unwired: 2 in, 2 out]
      n85 = property on="Master Data Material Description" class="Str"("Value"=w194) -> ()  [unwired: 2 in, 2 out]
    }
    frame "SELECT [ShortDescription]" {
      w305 = 1  # m.[MaterialRev]
      # "Copy MasterData.SAPMaterial: [MaterialNo],[ShortDescription] TO \nMasterData.Material: [MaterialNo],[Description]"
      n86 = Select(t="", s=w293, f="AND [Inactive] = '0'") -> (s? t:f=w298:string)
      n87 = call "DB - Replace DB.Schema.Table.vi"("DB.Schema.Table"=w286, "string in"="Use [<DB>]\n\nSELECT [ShortDescription] \nFROM [<Schema>].[<Table>] \n\nWHERE  [MaterialNo] = '<A>' AND [LanguageId] = '<L>' AND [Inactive] = '0' \n\n") -> ("string out"=w302:string)  [unwired: 8 in, 1 out]
      n88 = call "VI - Interactive or SubVI.vi"() -> ("Mode"=w292:T7)  [unwired: 5 in]
      n89 = Search and Replace String(replace all?=TRUE, input string=w302, search string="<A>", replace string=w299) -> (result string=w289:string)  [unwired: 4 in, 3 out]
      n90 = Search and Replace String(replace all?=TRUE, input string=w289, search string="<L>", replace string=w287) -> (result string=w288:string)  [unwired: 4 in, 3 out]
      n91 = Search and Replace String(input string=w288, search string="<AND>", replace string=w298) -> (result string=w295:string)  [unwired: 5 in, 3 out]
      n92 = call-poly <vilib>:"DB Tools Execute Query.vi"("error in (no error)"=w314, "SQL query"=w295, "connection reference"=w315) -> ("error out"=w310:errorcluster, "recordset reference"=w311:T11)  [unwired: 5 in]
      n93 = call-poly <vilib>:"DB Tools Fetch Recordset Data.vi"("error in (no error)"=w310, "recordset reference"=w311) -> ("error out"=w309:errorcluster, "recordset data"=w308:variant[][], "recordset reference out"=w306:T11)  [unwired: 3 in]
      n94 = xnode "Database Variant To Data"("database variant"=w308, "type"=string[][] []) -> ("data"=w284:string[][])  [unwired: 1 in, 1 out]
      n95 = Index Array(array=w284, index (row)=0, index (col)=0 ("disabled index (col)")) -> (element=w281:string)
      n96 = call-poly <vilib>:"DB Tools Free Object.vi"("error in (no error)"=w309, "recordset reference"=w306) -> ("error out"=w313:errorcluster)  [unwired: 8 in, 1 out]
      n97 = Index Array(array=w284, index (col)=w305) -> (element=w303:string[])  [unwired: 1 in]
      n98 = case shown="\"subVI Mode\"" w292 {
        tunnel: w304 -> [_ w323]
        tunnel: w303 -> [_ w322]
        tunnel: w285 -> [_ w320]
        tunnel: w281 -> [_ w316]
        frame "Interactive", Default {
          # "Not a Refnum"
        }
        frame "subVI Mode" {
          # "External Refnum connected"
          n99 = property class="Clust (strict)"(reference=w320) -> (reference out=w319:refnum<vi>, "Value"=w318:T3)  [unwired: 1 in, 1 out]
          n100 = Bundle By Name(cluster=w318, "Master Data Material Description"=w316) -> (w317:T3)
          n101 = property class="CmbBox"(reference=w323, "Strings[]"=w322) -> (error out=w321:errorcluster)  [unwired: 1 in, 1 out]
          n102 = local write "Property Node Error"(w321) -> ()
          n103 = property class="Clust (strict)"(reference=w319, "Value"=w317) -> ()  [unwired: 1 in, 2 out]
        }
      }
      n104 = property on="Master Data Rev" class="CmbBox"("Strings[]"=w303) -> ()  [unwired: 2 in, 2 out]
      n105 = property on="Master Data Material Description" class="Str"("Value"=w281) -> ()  [unwired: 2 in, 2 out]
    }
    frame "SELECT [Description], [ImageFile]" {
      w393 = 2  # [ImageFileName]
      w404 = 1  # [ImageFilePath]
      w411 = 3  # [Inactive]
      w412 = 0  # [Description]
      w394 = 0 ("disabled index (col)")
      n106 = case shown="True" w369 {
        tunnel: "Use [<DB>]\nSELECT  [Description]\n           ,[ImageFilePath]\n           ,[ImageFileName]\n           ,[Inactive]\n FROM \n[<Schema2>].[<Table2>] \n\nWHERE [MaterialNo] = '<M>' AND [MaterialRev] = '<R>'  AND [LanguageId] = '<L>' AND [Inactive] = '0' \n\n" -> [w420 w424]
        tunnel: [w420 w421] -> w368
        frame False {
        }
        frame True {
          n107 = Search and Replace String(input string=w424, search string="[Description]", replace string="CAST([Description] AS varbinary(max))") -> (result string=w421:string)  [unwired: 5 in, 3 out]
        }
      }
      n108 = call "DB - Replace DB.Schema.Table.vi"("DB.Schema.Table 2"=w376, "string in"=w368) -> ("string out"=w418:string)  [unwired: 8 in, 1 out]
      n109 = call "VI - Interactive or SubVI.vi"() -> ("Mode"=w392:T7)  [unwired: 5 in]
      n110 = property on="Material" class="Clust (strict)"() -> ("Value"=w408:T3)  [unwired: 2 in, 2 out]
      n111 = Search and Replace String(replace all?=TRUE ("replace all? (F)"), input string=w418, search string="<M>", replace string=w406) -> (result string=w417:string)  [unwired: 4 in, 3 out]
      n112 = Select(t="", s=w396, f="AND m.[Inactive] = '0' ") -> (s? t:f=w400:string)
      n113 = Search and Replace String(replace all?=TRUE ("replace all? (F)"), input string=w417, search string="<R>", replace string=w405) -> (result string=w380:string)  [unwired: 4 in, 3 out]
      n114 = Search and Replace String(replace all?=TRUE ("replace all? (F)"), input string=w380, search string="<L>", replace string=w378) -> (result string=w379:string)  [unwired: 4 in, 3 out]
      n115 = Search and Replace String(replace all?=FALSE ("replace all? (F)"), input string=w379, search string="<AND>", replace string=w400) -> (result string=w372:string)  [unwired: 4 in, 3 out]
      n116 = call "DB - T-SQL Query.vi"("error in (no error)"=w371, "T-SQL"=w372, "connection reference"=w373) -> ("error out"=w374:errorcluster, "2D data"=w375:string[][])  [unwired: 6 in, 1 out]
      n117 = Index Array(array=w375, index (row) #1=w394, index (col) #1=w412, index (row) #2=w394, index (col) #2=w411, index (row) #3=w394, index (col) #3=w404, index (row) #4=w394, index (col) #4=w393) -> (element #1=w402:string, element #2=w401:string, element #3=w388:string, element #4=w387:string)
      "ImageFileType" <- w387
      n118 = call "DB - Convert BIT Type.vi"("BIT Type (eg Inactive)"=w401) -> ("Boolean"=w403:bool)  [unwired: 2 in, 2 out]
      n119 = Empty String/Path?(string/path=w387) -> (empty?=w385:bool)
      n120 = Empty String/Path?(string/path=w388) -> (empty?=w386:bool)
      n121 = Not Or(1:w385, 2:w386) -> (0:w384:bool)
      n122 = String To Path(string=w388) -> (path=w391:path)
      n123 = Build Path(base path=w391, name or relative path=w387) -> (appended path=w390:path)
      "Material File" <- w390
      n124 = case shown="\"subVI Mode\"" w392 {
        tunnel: w409 -> [_ w447]
        tunnel: w402 -> [_ w446]
        tunnel: w403 -> [_ w445]
        tunnel: "Update [ShortDescription] to Cluster" -> [_ w444]
        frame "Interactive", Default {
          # "Not a Refnum"
        }
        frame "subVI Mode" {
          # "External Ref connected"
          n125 = property class="Clust (strict)"(reference=w447) -> (reference out=w443:refnum<vi>, "Value"=w449:T3)  [unwired: 1 in, 1 out]
          n126 = case shown="True" w444 {
            tunnel: w449 -> [w452 w456]
            tunnel: [w451 w455] -> w448
            tunnel: w446 -> [_ w454]
            tunnel: w445 -> [w450 w453]
            frame False {
              n127 = Bundle By Name(cluster=w452, "Inactive"=w450) -> (w451:T3)
            }
            frame True {
              n128 = Bundle By Name(cluster=w456, "Master Data Material Description"=w454, "Inactive"=w453) -> (w455:T3)
            }
          }
          n129 = property class="Clust (strict)"(reference=w443, "Value"=w448) -> ()  [unwired: 1 in, 2 out]
        }
      }
      n130 = case shown="True" w384 {
        tunnel: w390 -> [_ w437]
        tunnel: [w436 w441] -> w419
        tunnel: w374 -> [w436 w442]
        tunnel: [_ w439] -> w389
        tunnel: [_ w438] -> w383
        frame False {
        }
        frame True {
          # "Neither is Blank"
          n131 = call <vilib>:"Read JPEG File.vi"("error in (no error)"=w442, "path to JPEG file"=w437) -> ("error out"=w441:errorcluster, "image data"=w438:T1)  [unwired: 7 in, 1 out]
          "JPG File Error" <- w441
          n132 = Unbundle By Name(w441) -> ("status"=w440:bool)
          n133 = Not(x=w440) -> (.not. x?=w439:bool)
        }
      }
      "ImageFile OK" <- w389
      "image data" <- w383
      n134 = case shown="False" "Update [ShortDescription] to Cluster" {
        tunnel: w408 -> [w429 w435]
        tunnel: [w428 w434] -> w407
        tunnel: w406 -> [w427 w433]
        tunnel: w405 -> [w426 w432]
        tunnel: w403 -> [w425 w431]
        tunnel: w402 -> [_ w430]
        frame False {
          n135 = Bundle By Name(cluster=w429, "Master Data Material"=w427, "Master Data Rev"=w426, "Inactive"=w425) -> (w428:T3)
        }
        frame True {
          n136 = Bundle By Name(cluster=w435, "Master Data Material"=w433, "Master Data Rev"=w432, "Master Data Material Description"=w430, "Inactive"=w431) -> (w434:T3)
        }
      }
      n137 = Build Array(w402, w401) -> (w410:string[])
      n138 = property on="Material" class="Clust (strict)"("Value"=w407) -> ()  [unwired: 2 in, 2 out]
    }
  }
  "SUMMARY" <- w19
  "SQL Query" <- w19
  "SQL" <- w27
  "Results" <- w23
  n139 = flat-sequence {
    tunnel: [w457] -> w24
    frame #0 {
      n140 = Tick Count (ms)() -> (millisecond timer value=w457:u32)
    }
  }
  n141 = flat-sequence {
    tunnel: w19 -> [_]
    tunnel: w24 -> [w459]
    frame #0 {
      n142 = Tick Count (ms)() -> (millisecond timer value=w460:u32)
      n143 = Subtract(x=w460, y=w459) -> (x-y=→"ms":u32)
    }
  }
  n144 = case shown="True" w16 {
    tunnel: w7 -> [_ w462]
    tunnel: w19 -> [_ _]
    frame False {
    }
    frame True {
      n145 = call <vilib>:"DB Tools Close Connection.vi"("connection reference"=w462) -> ("error out"=→"Close Error":errorcluster)  [unwired: 6 in]
    }
  }
  n146 = global write "Global SRTRS.vi" "DB Error"(w19) -> ()
